vi "字符串数组转字符串.vi"(1 "号数数组":string[](array[string])) -> (0 "String":string)   [LabVIEW 2019]
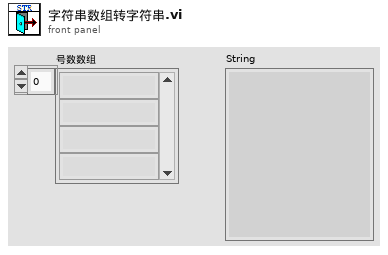
[diagram p1: front panel]
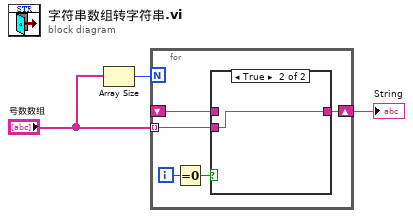
[diagram p0: block diagram]
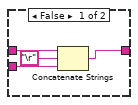
[diagram p2: hidden frame]
diagram:
  n1 = Array Size(array="号数数组") -> (size(s)=w3:i32)
  n2 = for {
    N: w3 -> [_]
    tunnel: "号数数组" -> [w6] mode=indexing
    shift-right: [w8] -> w1
    shift-left: _ -> [w7]
    i -> [w4]
    n3 = Equal To 0?(x=w4) -> (x = 0?=w5:bool)
    n4 = case shown="True" w5 {
      tunnel: [w11 w13] -> w8
      tunnel: w7 -> [w12 _]
      tunnel: w6 -> [w10 w13]
      frame False {
        n5 = Concatenate Strings(w12, "\r", w10) -> (w11:string)
      }
      frame True {
      }
    }
  }
  "String" <- w1
